vi "Read Attributes.vi"(11 "Fetch Rooms List and Size Limits Msg":refnum<class "Fetch Rooms List and Size Limits Msg.lvclass">) -> (2 "Payload":cluster{"Room Size":string})   [LabVIEW 2023, in "Guest Manager UI.lvlib" / "Fetch Rooms List and Size Limits Msg.lvclass"]
uses:
  Fetch Rooms List and Size Limits Msg.lvclass
  Fetch Rooms List and Size Limits Msg.lvclass/Fetch Rooms List and Size Limits Msg.ctl
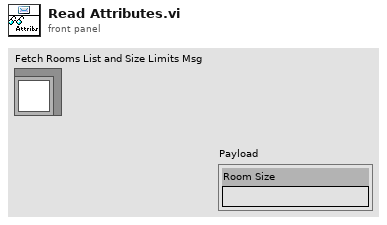
[diagram p1: front panel]
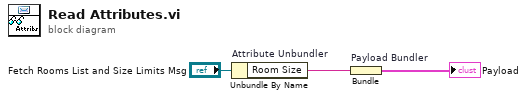
[diagram p0: block diagram]
diagram:
  n1 = Unbundle By Name "Attribute Unbundler"("Fetch Rooms List and Size Limits Msg") -> ("Room Size"=w1:string)
  n2 = Bundle "Payload Bundler"("Room Size"=w1) -> (→"Payload":cluster{"Room Size":string})  [unwired: 1 in]
